vi "VK-1701Edit Coating.vi"() -> ()   [LabVIEW 2009]
panel:
  out "Experiment_path":path
  out "Cancelled":bool
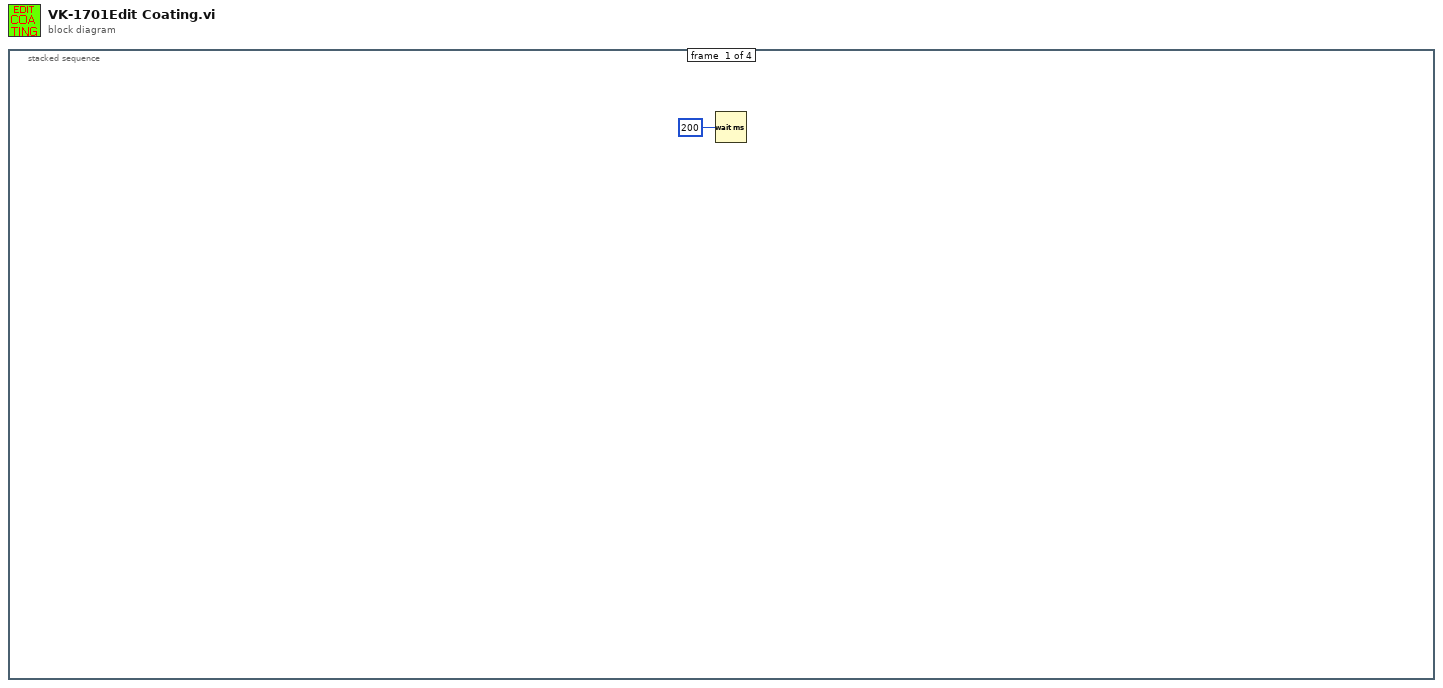
[diagram p0: block diagram]
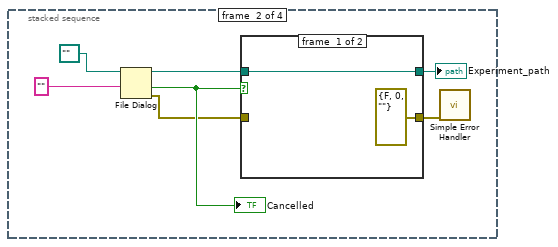
[diagram p2: hidden frame]
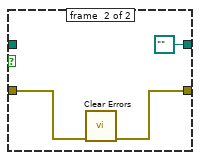
[diagram p3: hidden frame]
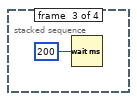
[diagram p4: hidden frame]
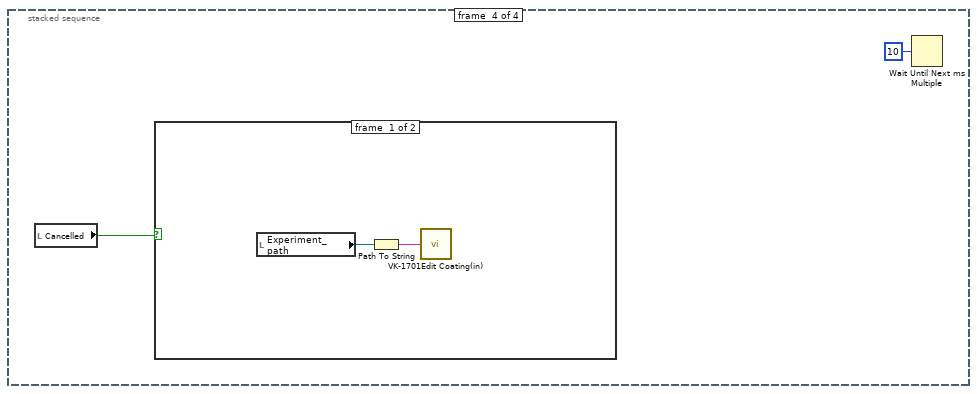
[diagram p5: hidden frame]
diagram:
  n1 = stacked-sequence {
    frame #0 {
      n2 = Wait (ms)(milliseconds to wait=u32 200) -> ()  [unwired: 1 out]
    }
    frame #1 {
      n3 = File Dialog(9:"" ("Path"), 11:path "" ("base path")) -> (0:w5:errorcluster, 1:w6:bool, 3:w4:path)  [unwired: 2 in, 4 out]
      "Cancelled" <- w6
      n4 = case shown="False" w6 {
        tunnel: w5 -> [_ w13]
        tunnel: [w10 path ""] -> w2
        tunnel: w4 -> [w10 _]
        tunnel: [errorcluster {"status"=FALSE, "code"=0, "source"=""} ("error out") w12] -> w3
        frame #0 {
        }
        frame #1 {
          n5 = call <vilib>:"Clear Errors.vi"("error in (no error)"=w13) -> ("error out"=w12:errorcluster)  [unwired: 6 in]
        }
      }
      "Experiment_path" <- w2
      n6 = call <vilib>:"Simple Error Handler.vi"("error in (no error)"=w3) -> ()  [unwired: 4 in, 5 out]
    }
    frame #2 {
      n7 = Wait (ms)(milliseconds to wait=u32 200) -> ()  [unwired: 1 out]
    }
    frame #3 {
      n8 = local read "Cancelled"() -> (w15:bool)
      n9 = case shown="False" w15 {
        frame #0 {
          n10 = local read "Experiment_path"() -> (w18:path)
          n11 = Path To String(path=w18) -> (string=w17:string)
          n12 = call "VK-1701Edit Coating(in).vi"("Path"=w17) -> ()
        }
        frame #1 {
        }
      }
      n13 = Wait Until Next ms Multiple(millisecond multiple=u32 10) -> ()  [unwired: 1 out]
    }
  }
